vi "Value.vi"(8 "error in (no error)":errorcluster, 11 "Literal in":refnum<class "Literal.lvclass">) -> (0 "error out":errorcluster, 2 "Value":i64, 3 "Literal out":refnum<class "Literal.lvclass">)   [LabVIEW 2020, in "Literal.lvclass"]
uses:
  Literal.lvclass
  Literal.lvclass/Literal.ctl
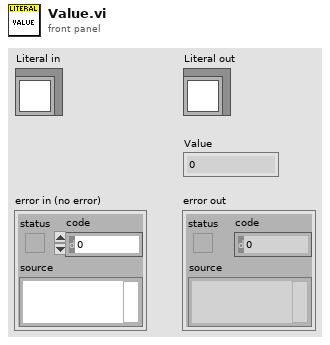
[diagram p1: front panel]
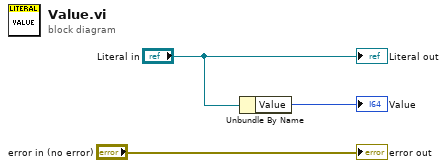
[diagram p0: block diagram]
diagram:
  n1 = Unbundle By Name("Literal in") -> ("Value"=→"Value":i32)
  "error out" <- "error in (no error)"
  "Literal out" <- "Literal in"
